vi "move85x(GPIB).vi"(0 "wait time(ms)":dbl=5000.0, 1 "Moving Distance (mm) : resolutino is 1um":dbl, 2 "Axis Number":u8, 3 "SHOT202 Address":string) -> ()   [LabVIEW 2010]
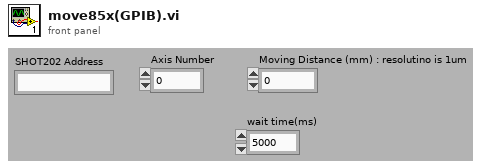
[diagram p1: front panel]
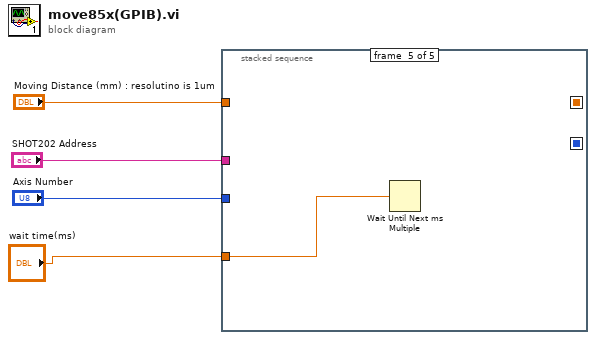
[diagram p0: block diagram]
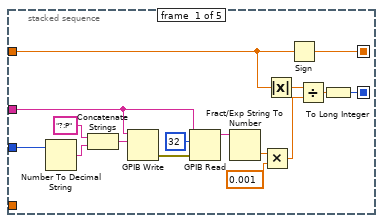
[diagram p2: hidden frame]
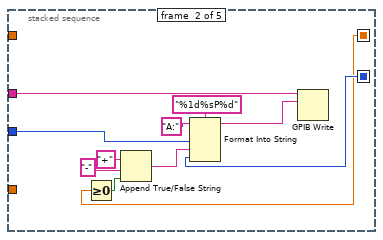
[diagram p3: hidden frame]
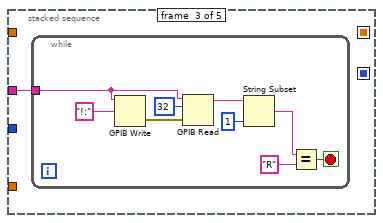
[diagram p4: hidden frame]
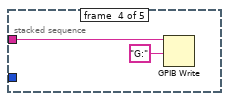
[diagram p5: hidden frame]
diagram:
  n1 = stacked-sequence {
    seq-local: [w12 _ _ _ _] -> [_ w21 _ _ _]
    seq-local: [w10 _ _ _ _] -> [_ w22 _ _ _]
    tunnel: "Axis Number" -> [w19 w28 _ _ _]
    tunnel: "SHOT202 Address" -> [w15 w25 w32 w43 _]
    tunnel: "Moving Distance (mm) : resolutino is 1um" -> [w6 _ _ _ _]
    tunnel: "wait time(ms)" -> [_ _ _ _ w44]
    frame #0 {
      n2 = Number To Decimal String(number=w19) -> (decimal integer string=w18:string)  [unwired: 1 in]
      n3 = Concatenate Strings("?:P" ("string"), w18) -> (w17:string)
      n4 = GPIB Write(0:w15, 1:w17) -> (6:w16:errorcluster)  [unwired: 3 in, 1 out]
      n5 = GPIB Read(0:w15, 1:32 ("byte count"), 3:w16) -> (5:w13:string)  [unwired: 2 in, 2 out]
      n6 = Fract/Exp String To Number(string=w13) -> (number=w9:dbl)  [unwired: 3 in, 1 out]
      n7 = Multiply(x=w9, y=0.001) -> (x*y=w8:dbl)
      n8 = Absolute Value(x=w6) -> (abs(x)=w7:dbl)
      n9 = Sign(1:w6) -> (0:w12:dbl)
      n10 = Divide(x=w7, y=w8) -> (x/y=w11:dbl)
      n11 = To Long Integer(number=w11) -> (32bit integer=w10:i32)
    }
    frame #1 {
      n12 = Greater Or Equal To 0?(x=w21) -> (x >= 0?=w23:bool)
      n13 = Append True/False String(1:w23, 2:"-", 3:"+") -> (0:w29:string)  [unwired: 1 in]
      n14 = Format Into String(format string="%1d%sP%d", initial string="A:", w28, w29, w22) -> (resulting string=w24:string)  [unwired: 1 in, 1 out]
      n15 = GPIB Write(0:w25, 1:w24) -> ()  [unwired: 3 in, 2 out]
    }
    frame #2 {
      n16 = while {
        tunnel: w32 -> [w40]
        stop <- w38 stop-if-true
        n17 = GPIB Write(0:w40, 1:"!:" ("data")) -> (6:w39:errorcluster)  [unwired: 3 in, 1 out]
        n18 = GPIB Read(0:w40, 1:32 ("byte count"), 3:w39) -> (5:w35:string)  [unwired: 2 in, 2 out]
        n19 = String Subset(string=w35, length (rest)=1 ("length (rest)")) -> (substring=w34:string)  [unwired: 1 in]
        n20 = Equal?(x=w34, y="R") -> (x = y?=w38:bool)
      }
    }
    frame #3 {
      n21 = GPIB Write(0:w43, 1:"G:" ("string")) -> ()  [unwired: 3 in, 2 out]
    }
    frame #4 {
      n22 = Wait Until Next ms Multiple(millisecond multiple=w44) -> ()  [unwired: 1 out]
    }
  }
